vi "waveform show.vi"(0 "curv array in":dbl[](array[numeric]), 2 "SW array in":dbl[](array[numeric]), 3 "Col Count 2":i16, 4 "coloumn curvness array":dbl[](array[numeric]), 5 "Sensor Pallet NUM 2":i16) -> ()   [LabVIEW 2019]
panel:
  out "Col Count":i16
  out "SideWall Sensors Graph":dynamicdata(graph)=[{"t0"=timestamp(3688782360.9322495 s since 1904-01-01), "dt"=1.0, "Y"=[6594.0]}, {"t0"=timestamp(3688782360.9322495 s since 1904-01-01), "dt"=1.0, "Y"=[65535.0]}]
  in  "Close Square":bool
  out "Col5 CURV(mm)":dbl format="%#.2g"
  out "Sensor Pallet NUM":i16
  out "Col1 CURV(mm)":dbl format="%#.2g"
  out "Col2 CURV(mm)":dbl format="%#.2g"
  out "Col3 CURV(mm)":dbl format="%#.2g"
  out "Col4 CURV(mm)":dbl format="%#.2g"
  out "Overal CURV(mm)":dbl format="%#.2g"
  out "Curvness Sensors Graph":dynamicdata(graph)
  # "DPIS"
  # "Sensor Trends"
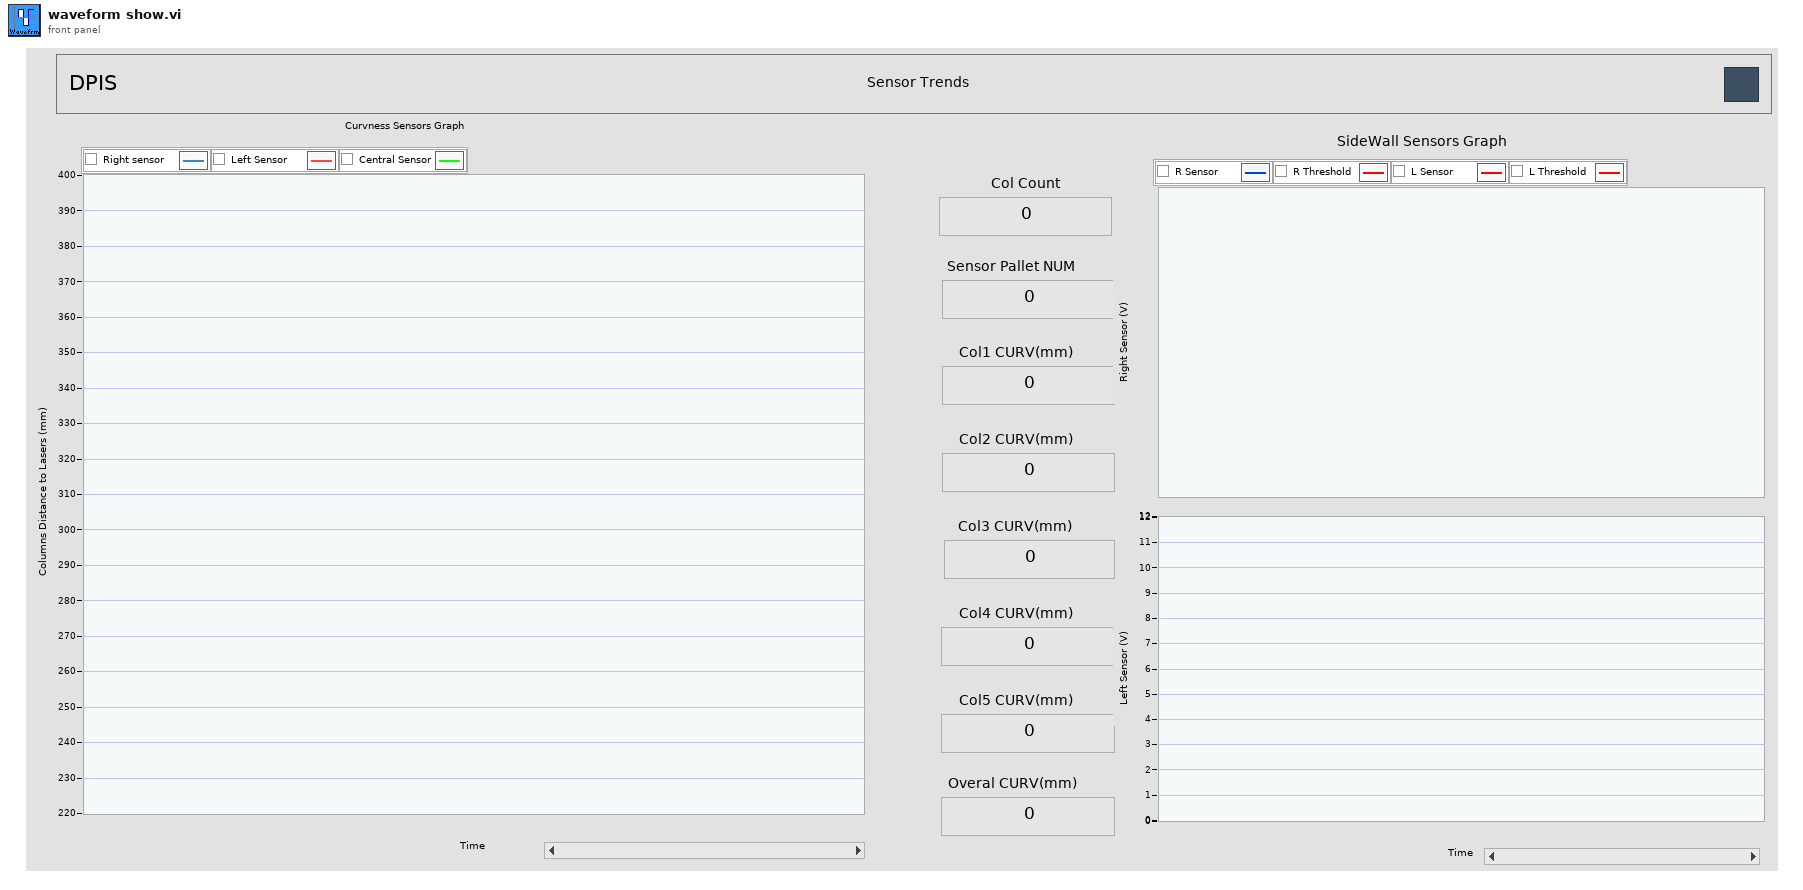
[diagram p1: front panel]
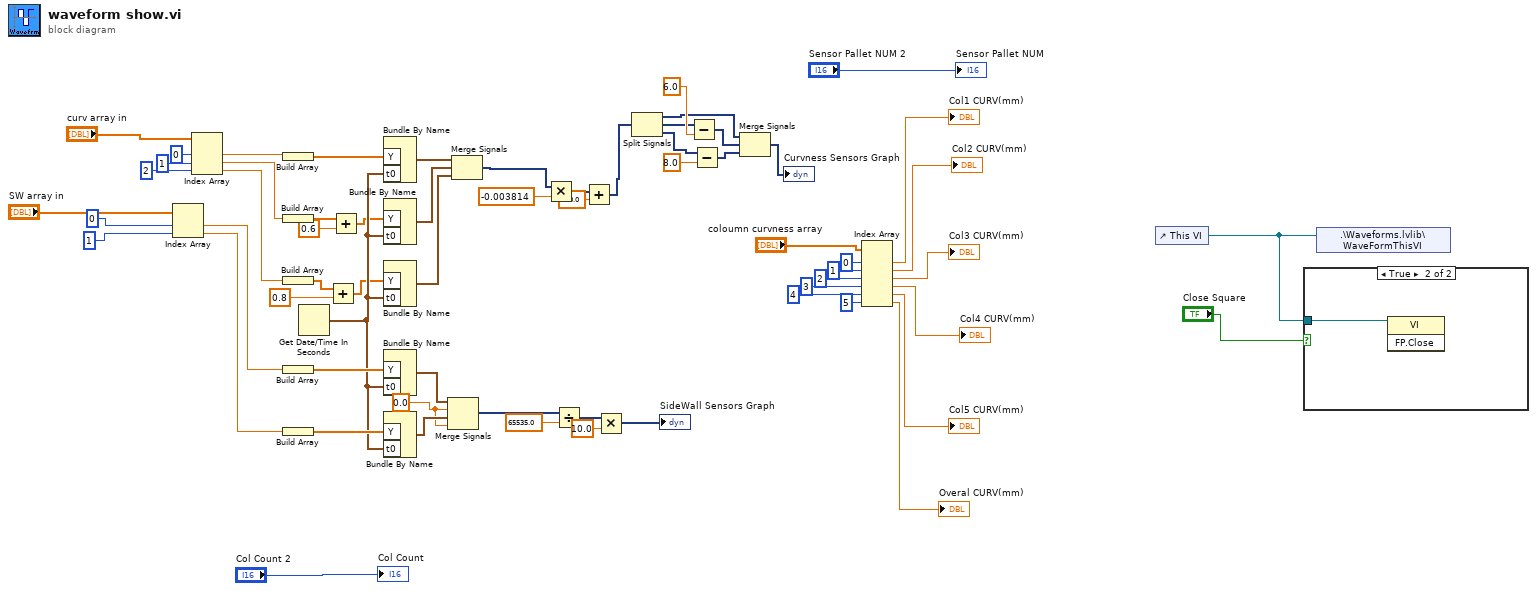
[diagram p0: block diagram]
diagram:
  w26 = 0.0
  n1 = Index Array(array="SW array in", index #1=0 ("index"), index #2=1 ("index")) -> (element #1=w45:dbl, element #2=w44:dbl)
  n2 = Index Array(array="curv array in", index #1=0 ("index"), index #2=1 ("index"), index #3=2 ("index")) -> (element #1=w56:dbl, element #2=w55:dbl, element #3=w54:dbl)
  n3 = Build Array(w56) -> (w61:dbl[])
  n4 = Build Array(w55) -> (w15:dbl[])
  n5 = Build Array(w54) -> (w18:dbl[])
  n6 = Build Array(w45) -> (w52:dbl[])
  n7 = Build Array(w44) -> (w53:dbl[])
  n8 = Get Date/Time In Seconds() -> (seconds since 1Jan1904=w51:timestamp)
  n9 = Add(x=w18, y=0.8) -> (x+y=w17:dbl[])
  n10 = Add(x=w15, y=0.6) -> (x+y=w14:dbl[])
  n11 = Bundle By Name("Y"=w61, "t0"=w51) -> (w60:waveform(dbl))  [unwired: 1 in]
  n12 = Bundle By Name("Y"=w14, "t0"=w51) -> (w63:waveform(dbl))  [unwired: 1 in]
  n13 = Bundle By Name("Y"=w17, "t0"=w51) -> (w62:waveform(dbl))  [unwired: 1 in]
  n14 = Bundle By Name("Y"=w52, "t0"=w51) -> (w50:waveform(dbl))  [unwired: 1 in]
  n15 = Bundle By Name("Y"=w53, "t0"=w51) -> (w27:waveform(dbl))  [unwired: 1 in]
  n16 = Merge Signals(w50, w26, w27, w26) -> (w21:dynamicdata)
  n17 = Merge Signals(w60, w63, w62) -> (w4:dynamicdata)
  n18 = Multiply(x=w4, y=-0.003814) -> (x*y=w3:dynamicdata)
  n19 = Divide(x=w21, y=65535.0) -> (x/y=w23:dynamicdata)
  n20 = Add(x=w3, y=400.0) -> (x+y=w1:dynamicdata)
  n21 = Multiply(x=w23, y=10.0) -> (x*y=→"SideWall Sensors Graph":dynamicdata)
  n22 = Split Signals(w1) -> (w8:dynamicdata, w12:dynamicdata, w10:dynamicdata)  [unwired: 3 in]
  n23 = Subtract(x=w12, y=6.0) -> (x-y=w7:dynamicdata)
  n24 = Subtract(x=w10, y=8.0) -> (x-y=w9:dynamicdata)
  n25 = Merge Signals(w8, w7, w9) -> (→"Curvness Sensors Graph":dynamicdata)
  n26 = Index Array(array="coloumn curvness array", index #1=0 ("index"), index #2=1 ("index"), index #3=2 ("index"), index #4=3 ("index"), index #5=4 ("index"), index #6=5 ("index")) -> (element #1=→"Col1 CURV(mm)":dbl, element #2=→"Col2 CURV(mm)":dbl, element #3=→"Col3 CURV(mm)":dbl, element #4=→"Col4 CURV(mm)":dbl, element #5=→"Col5 CURV(mm)":dbl, element #6=→"Overal CURV(mm)":dbl)
  n27 = control-ref of="This VI"() -> (w31:refnum<vi>)
  n28 = case shown="True" "Close Square" {
    tunnel: w31 -> [_ w64]
    frame False {
    }
    frame True {
      n29 = invoke class="VI" method="FP.Close"(reference=w64) -> ()  [unwired: 2 in, 3 out]
    }
  }
  n30 = shared-variable ".\\Waveforms.lvlib\\WaveFormThisVI"(w31) -> ()  [unwired: 1 in, 1 out]
  "Sensor Pallet NUM" <- "Sensor Pallet NUM 2"
  "Col Count" <- "Col Count 2"
